vi "Apply Motor Angle.vi"(9 "ccw angle offset (rad)":fxp<+/-,32,4>, 10 "ccw angle (rad)":fxp<+/-,32,4>, 11 "digital output line":refnum<k21>="Port0/DIO0") -> ()   [LabVIEW 2013, in "NI_Robotics_Hitec HS400 Series (FPGA).lvlib"]
doc: "Applies the motor angle in rad."
uses:
  NI_Robotics_Hitec HS400 Series (FPGA).lvlib
  <vilib>/robotics/Utilities/FPGA Utilities/Generate Digital Pulse (uSec).vi
  <vilib>/robotics/Utilities/FPGA Utilities/NI_Robotics_FPGA Utilities.lvlib
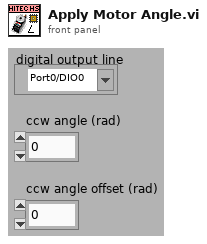
[diagram p1: front panel]
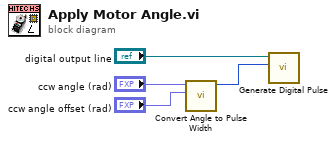
[diagram p0: block diagram]
diagram:
  n1 = call "Convert Angle to Pulse Width.vi"("ccw angle offset (rad)"="ccw angle offset (rad)", "ccw angle (rad)"="ccw angle (rad)") -> ("pulse width (uSec)"=w1:u32)  [unwired: 9 in]
  n2 = call-poly <vilib>:"Generate Digital Pulse.vi"("pulse width (uSec)"=w1, "FPGA digital output"="digital output line") -> ()  [unwired: 10 in]
